vi "Image_Pixel_Values_RE_GCFS.vi"(4 "date/time string":string, 5 "Image in":T3, 6 "Temperature":dbl format="%#_13g", 7 "Cluster":T1={"Core"={"Current VI Reference"=refnum, "Close Panel on Exit?"=FALSE}, "Your Boolean data"=FALSE, "Your string data"="", "Camera Cluster"={"Session"="", "Image"=refnum, "Position Image"=refnum, "PixelVal Image"=refnum, "Position Image Rings"=refnum, "Lable Image"=refnum, "Merged Image"=refnum}, "Data In Cluster"={"Images"={"Position Image path"=path "", "Sample folder path"=path "", "Rerun Folder path"=path "", "Rerun pos.img. path"=path ""}, "Sample Name"="", "Rerun Time"="", "Freezing value"=250.0, "Number of images"=0, "Overlay"=[]}, "Active"=FALSE, "Ready"=FALSE, "Exit"=FALSE, "Program_Start"="", "Data Out Cluster"={"Particle Measurements"=[], "Number of droplets"=0, "Time and temp"=[], "Sample time (YYYY-MM-DD_hh;mm)"=""}, "Load Rerun"=FALSE, "Rerun"=FALSE} {"Data Out Cluster"."Particle Measurements" format="%.2f"}) -> (0 "error out":errorcluster, 1 "Value_Array":string[](array[string]), 2 "Freezing_points":string[](array[string]), 3 "Freezing data":bool)   [LabVIEW 2024]
uses:
  <vilib>/vision/Image Controls.llb/IMAQ Image.ctl
  RerunCluster_GCFS.ctl
  <vilib>/userDefined/High Color/IMAQdx.ctl
  <vilib>/regexp/Match Regular Expression.xnode
  <vilib>/vision/NI_Vision_Development_Module.lvlib
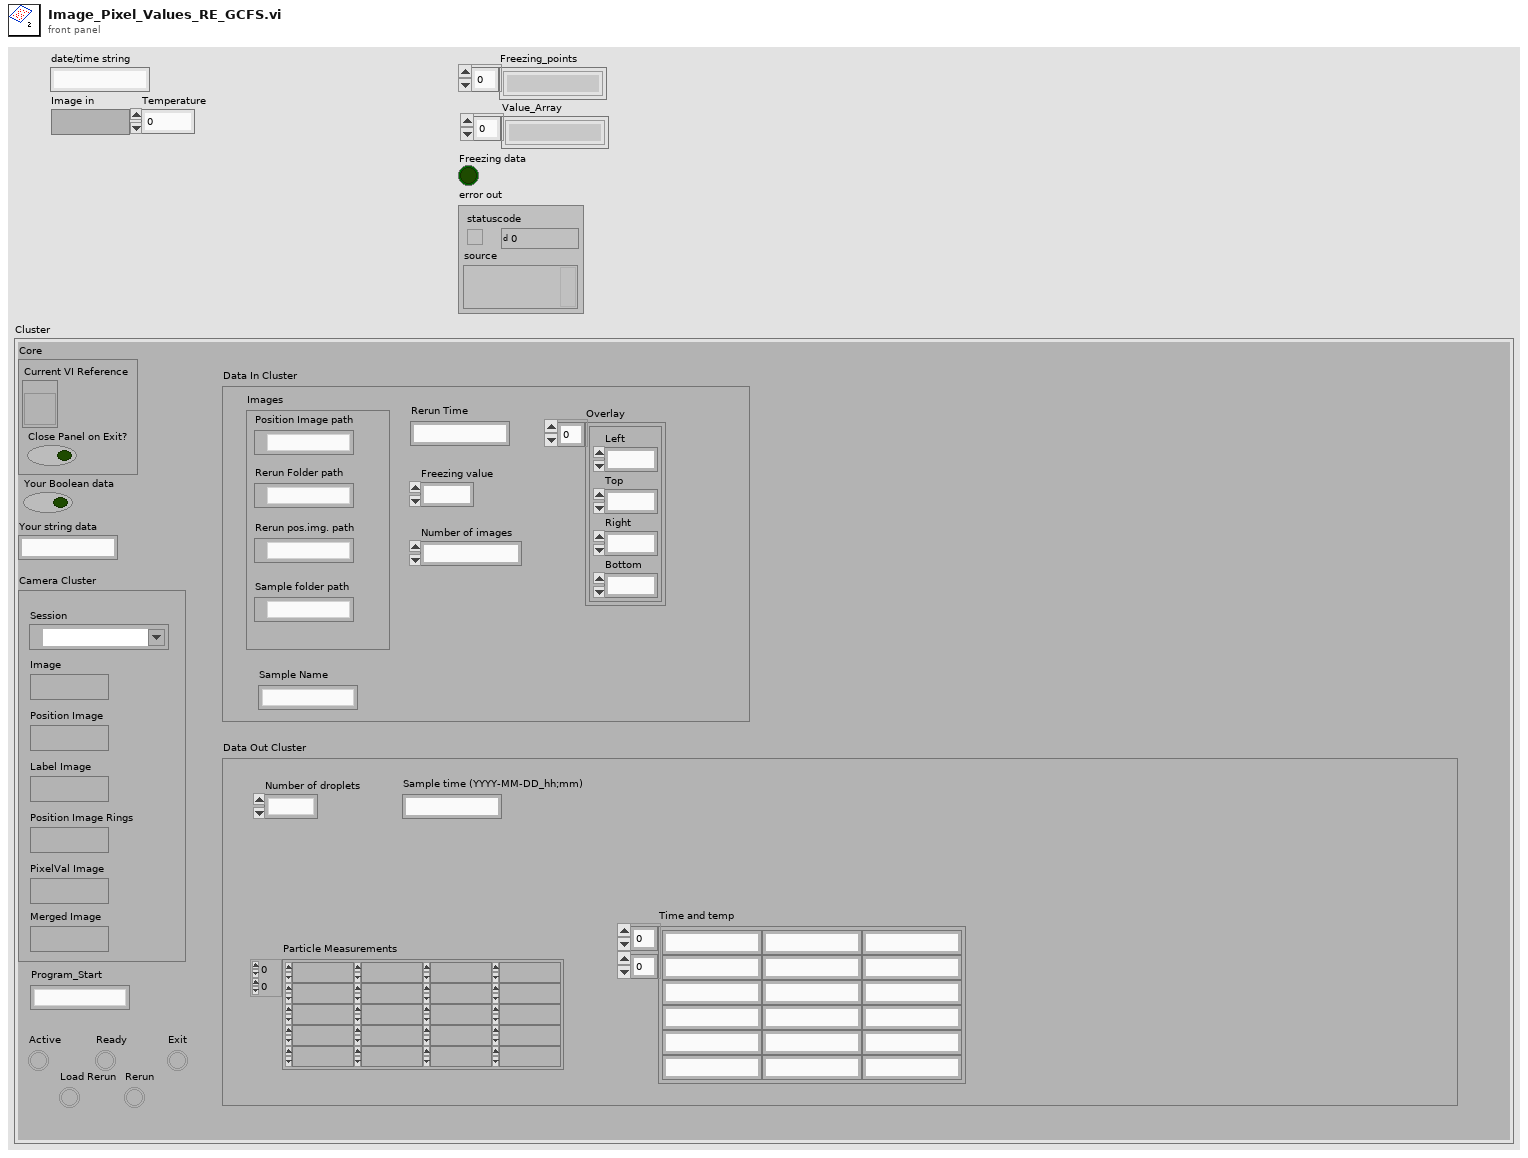
[diagram p1: front panel]
types:
  T1 = typedef "RerunCluster_GCFS.ctl" = cluster{"Core":cluster{"Current VI Reference":refnum<vi>, "Close Panel on Exit?":bool}, "Your Boolean data":bool, "Your string data":string, "Camera Cluster":cluster{"Session":T2, "Image":T3, "Position Image":T3, "PixelVal Image":T3, "Position Image Rings":T3, "Lable Image":T3, "Merged Image":T3}, "Data In Cluster":cluster{"Images":cluster{"Position Image path":path, "Sample folder path":path, "Rerun Folder path":path, "Rerun pos.img. path":path}, "Sample Name":string, "Rerun Time":string, "Freezing value":sgl, "Number of images":i32, "Overlay":cluster{"Left":i32, "Top":i32, "Right":i32, "Bottom":i32}[]}, "Active":bool, "Ready":bool, "Exit":bool, "Program_Start":string, "Data Out Cluster":cluster{"Particle Measurements":dbl[][], "Number of droplets":i32, "Time and temp":string[][], "Sample time (YYYY-MM-DD_hh;mm)":string}, "Load Rerun":bool, "Rerun":bool}
  T2 = typedef "IMAQdx.ctl" = refnum<k21>
  T3 = typedef "IMAQ Image.ctl" = refnum<image>
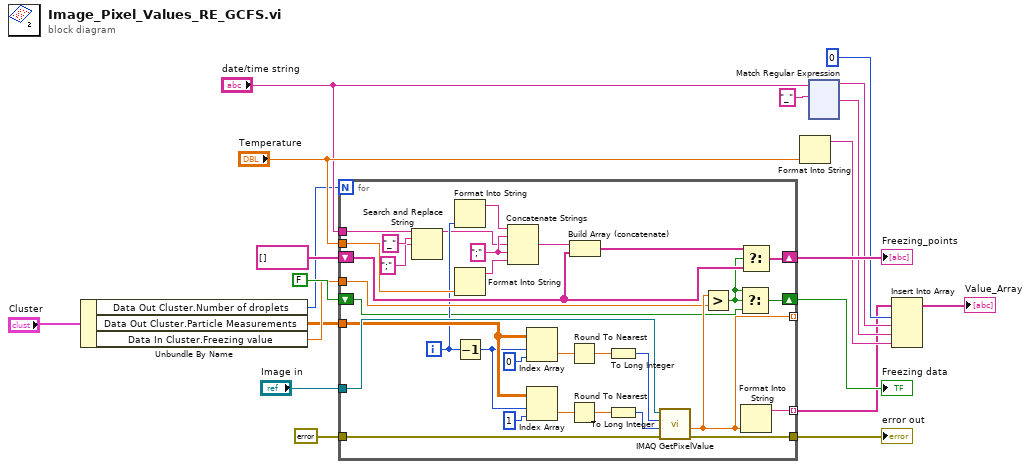
[diagram p0: block diagram]
diagram:
  n1 = Unbundle By Name("Cluster") -> ("Data Out Cluster.Number of droplets"=w3:i32, "Data Out Cluster.Particle Measurements"=w4:dbl[][], "Data In Cluster.Freezing value"=w5:sgl)
  n2 = for {
    N: w3 -> [_]
    tunnel: "Image in" -> [w52]
    tunnel: [w48] -> _ mode=indexing
    tunnel: [w49] -> w10 mode=indexing
    tunnel: "date/time string" -> [w24]
    shift-right: [w47] -> w19
    shift-left: string[] [] -> [w43]
    tunnel: w5 -> [w42]
    tunnel: "Temperature" -> [w40]
    tunnel: w4 -> [w36]
    shift-right: [w28] -> w17
    shift-left: FALSE -> [w27]
    tunnel: errorcluster {"status"=FALSE, "code"=0, "source"=""} ("error in (no error)") -> [w26]
    tunnel: [w25] -> w6
    i -> [w35]
    w41 = ";" ("string")
    n3 = Search and Replace String(input string=w24, search string="_" ("input string"), replace string=";" ("replace string (\"\")")) -> (result string=w23:string)  [unwired: 5 in, 3 out]
    n4 = Format Into String(w35) -> (resulting string=w46:string)  [unwired: 3 in, 1 out]
    n5 = Format Into String(w40) -> (resulting string=w39:string)  [unwired: 3 in, 1 out]
    n6 = Decrement(x=w35) -> (x-1=w34:i32)
    n7 = Concatenate Strings(w46, w41, w23, w41, w39) -> (w45:string)
    n8 = Index Array(array=w36, index (row)=w34, index (col)=0 ("disabled index (col)")) -> (element=w30:dbl)
    n9 = Index Array(array=w36, index (row)=w34, index (col)=1) -> (element=w33:dbl)
    n10 = Round To Nearest(number=w30) -> (nearest integer value=w31:dbl)
    n11 = Round To Nearest(number=w33) -> (nearest integer value=w32:dbl)
    n12 = Build Array (concatenate)(w45, w43) -> (w44:string[])
    n13 = To Long Integer(number=w31) -> (32bit integer=w51:i32)
    n14 = To Long Integer(number=w32) -> (32bit integer=w50:i32)
    n15 = call "IMAQ GetPixelValue"("Image"=w52, "X Coordinate"=w51, "Y Coordinate"=w50, "error in (no error)"=w26) -> ("Pixel Value (Float)"=w48:sgl, "error out"=w25:errorcluster)  [unwired: 2 in, 3 out]
    n16 = Greater?(x=w48, y=w42) -> (0:w29:bool)
    n17 = Select(t=w29, s=w29, f=w27) -> (s? t:f=w28:bool)
    n18 = Select(t=w44, s=w29, f=w43) -> (s? t:f=w47:string[])
    n19 = Format Into String(w48) -> (resulting string=w49:string)  [unwired: 3 in, 1 out]
  }
  "Freezing_points" <- w19
  "Freezing data" <- w17
  "error out" <- w6
  n20 = Format Into String("Temperature") -> (resulting string=w11:string)  [unwired: 3 in, 1 out]
  n21 = xnode "Match Regular Expression"("input string"="date/time string", "regular expression"="_" ("search string/char (-)")) -> ("before match"=w12:string, "after match"=w13:string)  [unwired: 4 in, 3 out]
  n22 = Insert Into Array(array=w10, index=0, new element #1=w12, new element #2=w13, new element #3=w11) -> (→"Value_Array":string[])
